vi "IMAQ FPGA CXP Pixel Buffer 8-Bit x 16.vi"(7 "Reset":bool, 8 "Read":bool, 9 "Tap":u8=8, 10 "Valid Bytes":u8, 11 "Pixel Data In U8x32":u8[](array[numeric])=[0, 0, 0, 0, 0, 0, 0, 0, 0, 0, 0, 0, 0, 0, 0, 0, 0, 0, 0, 0, 0, 0, 0, 0, 0, 0, 0, 0, 0, 0, 0, 0]) -> (2 "#Elements Read":u8, 3 "Pixel Data Out U8x8":u8[](array[numeric]))   [LabVIEW 2020]
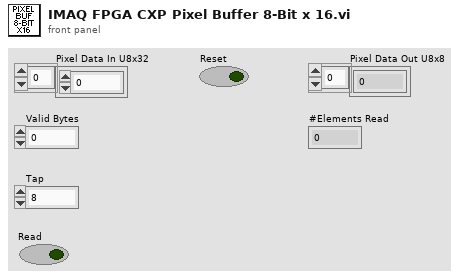
[diagram p1: front panel]
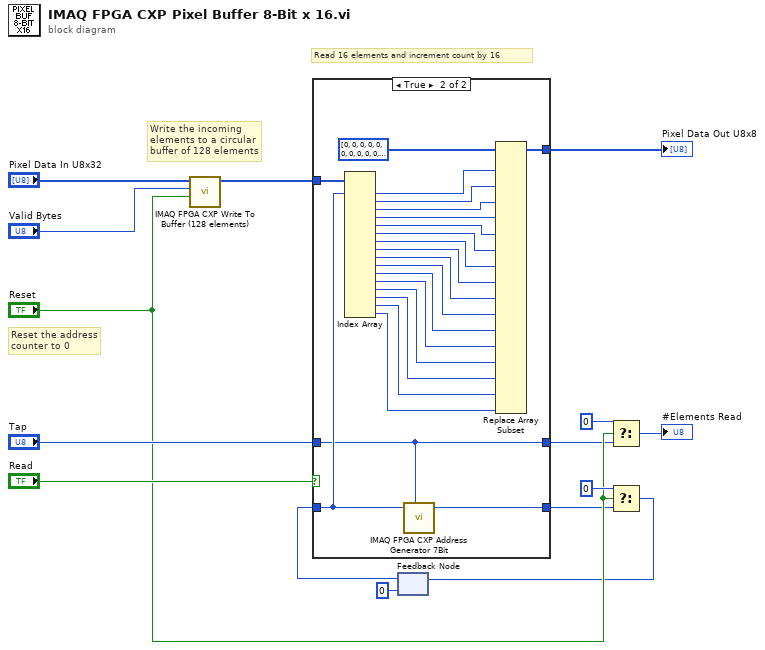
[diagram p0: block diagram]
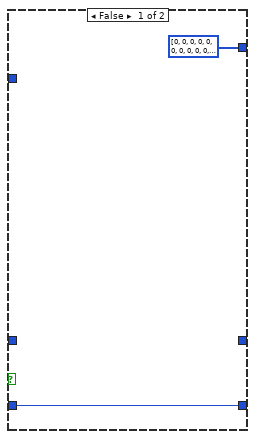
[diagram p2: hidden frame]
diagram:
  # "Reset the address\ncounter to 0"
  # "Write the incoming\nelements to a circular\nbuffer of 128 elements"
  # "Read 16 elements and increment count by 16"
  n1 = call <vilib>:"IMAQ FPGA CXP Write To Buffer (128 elements).vi"("Reset"="Reset", "Valid Bytes"="Valid Bytes", "Pixel Data In U8x32"="Pixel Data In U8x32") -> ("Buffer Out"=w8:u8[])  [unwired: 8 in]
  n2 = feedback #1(u8 0 ("y")) -> (w14:u8)
  n3 = case shown="True" "Read" {
    tunnel: w8 -> [_ w39]
    tunnel: [_ w27] -> w4
    tunnel: [u8[] [0, 0, 0, 0, 0, 0, 0, 0, 0, 0, 0, 0, 0, 0, 0, 0] w37] -> w13
    tunnel: [w17 w26] -> w3
    tunnel: w14 -> [w17 w28]
    tunnel: "Tap" -> [_ w27]
    frame False {
    }
    frame True {
      n4 = Index Array(array=w39, index #1=w28) -> (element #1=w36:u8, element #2=w35:u8, element #3=w34:u8, element #4=w33:u8, element #5=w32:u8, element #6=w31:u8, element #7=w30:u8, element #8=w29:u8, element #9=w25:u8, element #10=w24:u8, element #11=w23:u8, element #12=w22:u8, element #13=w21:u8, element #14=w20:u8, element #15=w19:u8, element #16=w18:u8)  [unwired: 15 in]
      n5 = call <vilib>:"IMAQ FPGA CXP Address Generator 7Bit.vi"("Base Address"=w28, "Index"=w27) -> ("Address Out"=w26:u8)  [unwired: 7 in]
      n6 = Replace Array Subset(array=u8[] [0, 0, 0, 0, 0, 0, 0, 0, 0, 0, 0, 0, 0, 0, 0, 0], new element #1=w36, new element #2=w35, new element #3=w34, new element #4=w33, new element #5=w32, new element #6=w31, new element #7=w30, new element #8=w29, new element #9=w25, new element #10=w24, new element #11=w23, new element #12=w22, new element #13=w21, new element #14=w20, new element #15=w19, new element #16=w18) -> (w37:u8[])  [unwired: 16 in]
    }
  }
  "Pixel Data Out U8x8" <- w13
  n7 = Select(t=u8 0 ("Tap"), s="Reset", f=w4) -> (s? t:f=→"#Elements Read":u8)
  n8 = Select(t=u8 0 ("y"), s="Reset", f=w3) -> (s? t:f=w2:u8)
  n9 = feedback-in #1(w2) -> ()
